vi "6220.vi"(2 "率":dbl=10.0, 3 "采样数":i32=10, 4 "timeout (s)":dbl=10.0 caption="超时(s)" format="%0.2f", 5 "error in":errorcluster caption="错误输入", 7 "stop (F)":bool caption="停止(F)", 10 "设备名":tag="PXI1Slot2") -> (14 "task out":refnum<k21> caption="任务输出", 15 "6220":cluster{"时间":timestamp, "数据":sgl[][]}, 18 "stopped":bool caption="已停止", 19 "error out":errorcluster caption="错误输出")   [LabVIEW 2014]
doc: "通过NI-DAQmx创建、编辑和运行任务。关于NI-DAQmx支持设备的完整列表，见NI-DAQ自述文件。\n\n在程序框图上放置DAQ助手Express VI，可通过DAQ助手新建任务。创建任务后，双击DAQ助手Express VI可编辑该任务。如需连续进行测量或信号生成，可将DAQ助手Express VI置于While循环内。"
uses:
  <vilib>/DAQmx/read.llb/DAQmx Read.vi
  <vilib>/DAQmx/read.llb/DAQmx Read (Analog 2D DBL NChan NSamp).vi
  <vilib>/DAQmx/miscellaneous.llb/DAQmx Fill In Error Info.vi
  <vilib>/DAQmx/configure/timing.llb/DAQmx Timing (Sample Clock).vi
  <vilib>/DAQmx/create/channels.llb/DAQmx Create Channel (AI-Voltage-Basic).vi
  <vilib>/DAQmx/create/channels.llb/DAQmx Create Channel (TEDS-AI-Voltage-Basic).vi
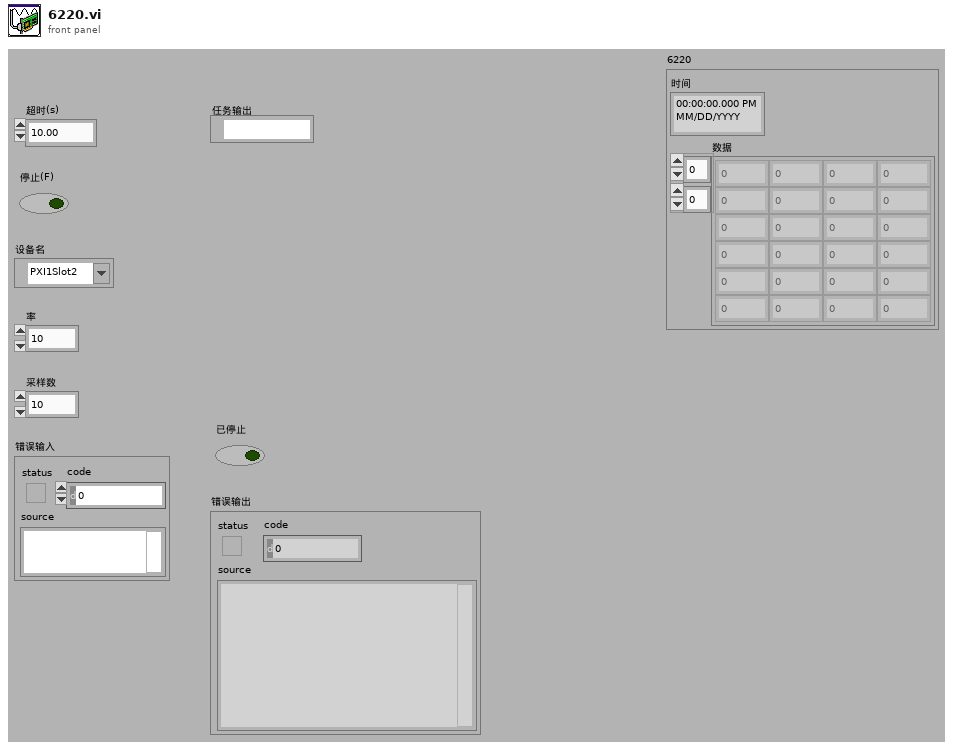
[diagram p1: front panel]
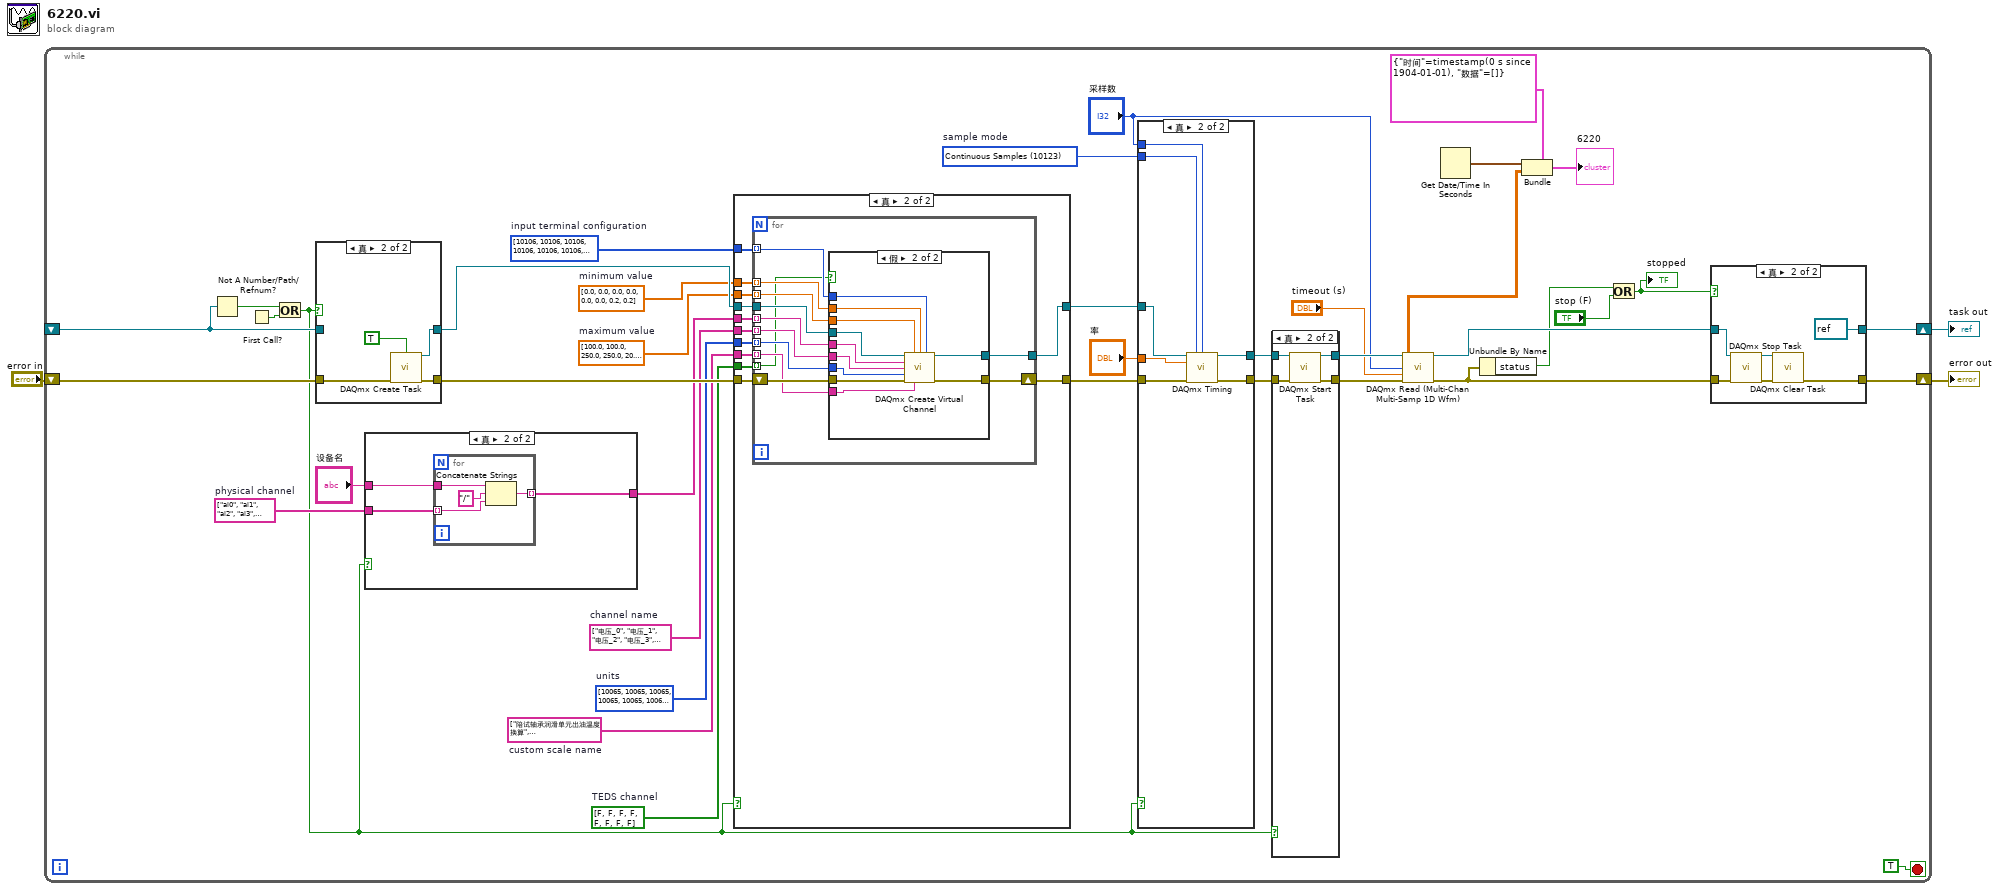
[diagram p0: block diagram]
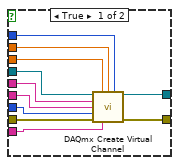
[diagram p6: hidden frame]
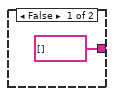
[diagram p7: hidden frame]
diagram:
  n1 = while {
    shift-right: [w14] -> w1
    shift-left: _ -> [w39]
    shift-right: [w12] -> w2
    shift-left: "error in" -> [w40]
    stop <- TRUE stop-if-true
    w22 = 10123 items=["Finite Samples"=10178, "Continuous Samples"=10123, "Hardware Timed Single Point"=12522]  # sample mode
    w26 = bool[] [FALSE, FALSE, FALSE, FALSE, FALSE, FALSE, FALSE, FALSE]  # TEDS channel
    w27 = string[] ["陪试轴承润滑单元出油温度换算", "陪试轴承润滑单元出油温度换算", "轴承外圈温度换算", "轴承外圈温度换算", "摩擦力换算", "摩擦力换算", "油缸力换算", "油缸力换算"]  # custom scale name
    w28 = i32[] [10065, 10065, 10065, 10065, 10065, 10065, 10065, 10065] items=["Volts"=10348, "From TEDS"=12516, "From Custom Scale"=10065]  # units
    w29 = string[] ["电压_0", "电压_1", "电压_2", "电压_3", "电压_4", "电压_5", "电压_6", "电压_7"]  # channel name
    w31 = dbl[] [100.0, 100.0, 250.0, 250.0, 20.0, 20.0, 7.0, 7.0]  # maximum value
    w32 = dbl[] [0.0, 0.0, 0.0, 0.0, 0.0, 0.0, 0.2, 0.2]  # minimum value
    w33 = i32[] [10106, 10106, 10106, 10106, 10106, 10106, 10106, 10106] items=["default"=-1, "RSE"=10083, "NRSE"=10078, "Differential"=10106, "Pseudodifferential"=12529]  # input terminal configuration
    w36 = string[] ["ai0", "ai1", "ai2", "ai3", "ai4", "ai5", "ai6", "ai7"]  # physical channel
    n2 = Not A Number/Path/Refnum?(number/path/refnum=w39) -> (NaN/Path/Refnum?=w38:bool)
    n3 = First Call?() -> (First Call?: T/F=w41:bool)
    n4 = Or(x=w38, y=w41) -> (x .or. y?=w21:bool)
    n5 = case "条件结构" shown="真" w21 {
      tunnel: [w123 w127] -> w35
      tunnel: w39 -> [w123 _]
      tunnel: [w122 w126] -> w34
      tunnel: w40 -> [w122 w124]
      frame False {
      }
      frame True {
        n6 = call <vilib>:"DAQmx Create Task.vi"("auto cleanup"=TRUE, "error in"=w124) -> ("task out"=w127:refnum<k21>, "error out"=w126:errorcluster)  [unwired: 12 in]
      }
    }
    n7 = case "条件结构" shown="真" w21 {
      tunnel: [string[] [] w117] -> w30
      tunnel: "设备名" -> [_ w116]
      tunnel: w36 -> [_ w115]
      frame False {
      }
      frame True {
        n8 = for "For循环" {
          tunnel: [w121] -> w117 mode=indexing
          tunnel: w116 -> [w120]
          tunnel: w115 -> [w118] mode=indexing
          n9 = Concatenate Strings(w120, "/" ("string"), w118) -> (w121:string)
        }
      }
    }
    n10 = case "条件结构" shown="真" w21 {
      tunnel: [w67 w77] -> w25
      tunnel: w35 -> [w67 w79]
      tunnel: [w66 w76] -> w24
      tunnel: w34 -> [w66 w78]
      tunnel: w33 -> [_ w75]
      tunnel: w32 -> [_ w74]
      tunnel: w31 -> [_ w73]
      tunnel: w30 -> [_ w72]
      tunnel: w29 -> [_ w71]
      tunnel: w28 -> [_ w70]
      tunnel: w27 -> [_ w69]
      tunnel: w26 -> [_ w68]
      frame False {
      }
      frame True {
        n11 = for "For循环" {
          tunnel: w79 -> [w91]
          tunnel: [w89] -> w77
          tunnel: w75 -> [w87] mode=indexing
          tunnel: w74 -> [w86] mode=indexing
          tunnel: w73 -> [w85] mode=indexing
          tunnel: w72 -> [w84] mode=indexing
          tunnel: w71 -> [w83] mode=indexing
          tunnel: w70 -> [w82] mode=indexing
          tunnel: w69 -> [w81] mode=indexing
          shift-right: [w88] -> w76
          shift-left: w78 -> [w90]
          tunnel: w68 -> [w80] mode=indexing
          n12 = case "条件结构" shown="假" w80 {
            tunnel: w91 -> [w102 w113]
            tunnel: w90 -> [w101 w112]
            tunnel: [w100 w111] -> w89
            tunnel: [w99 w110] -> w88
            tunnel: w87 -> [w98 w109]
            tunnel: w86 -> [w97 w108]
            tunnel: w85 -> [w96 w107]
            tunnel: w84 -> [w95 w106]
            tunnel: w83 -> [w94 w105]
            tunnel: w82 -> [w93 w104]
            tunnel: w81 -> [w92 w103]
            frame True {
              n13 = call-poly <vilib>:"DAQmx Create Virtual Channel.vi"("task in"=w102, "maximum value"=w96, "minimum value"=w97, "input terminal configuration"=w98, "physical channels"=w95, "name to assign"=w94, "units"=w93, "error in"=w101, "custom scale name"=w92) -> ("task out"=w100:refnum<k21>, "error out"=w99:errorcluster)  [unwired: 5 in]
            }
            frame False {
              n14 = call-poly <vilib>:"DAQmx Create Virtual Channel.vi"("task in"=w113, "maximum value"=w107, "minimum value"=w108, "input terminal configuration"=w109, "physical channels"=w106, "name to assign"=w105, "units"=w104, "error in"=w112, "custom scale name"=w103) -> ("task out"=w111:refnum<k21>, "error out"=w110:errorcluster)  [unwired: 5 in]
            }
          }
        }
      }
    }
    n15 = case "条件结构" shown="真" w21 {
      tunnel: [w58 w60] -> w20
      tunnel: w25 -> [w58 w63]
      tunnel: [w57 w59] -> w19
      tunnel: w24 -> [w57 w61]
      tunnel: "采样数" -> [_ w65]
      tunnel: w22 -> [_ w64]
      tunnel: "率" -> [_ w62]
      frame False {
      }
      frame True {
        n16 = call-poly <vilib>:"DAQmx Timing.vi"("task/channels in"=w63, "sample mode"=w64, "samples per channel"=w65, "rate"=w62, "error in"=w61) -> ("task out"=w60:refnum<k21>, "error out"=w59:errorcluster)  [unwired: 9 in]
      }
    }
    n17 = case "条件结构" shown="真" w21 {
      tunnel: [w52 w55] -> w18
      tunnel: w20 -> [w52 w56]
      tunnel: [w51 w53] -> w17
      tunnel: w19 -> [w51 w54]
      frame False {
      }
      frame True {
        n18 = call <vilib>:"DAQmx Start Task.vi"("task/channels in"=w56, "error in"=w54) -> ("task out"=w55:refnum<k21>, "error out"=w53:errorcluster)  [unwired: 12 in]
      }
    }
    n19 = call-poly "DAQmx Read (Multi-Chan Multi-Samp 1D Wfm).vi"("task/channels in"=w18, "number of samples per channel"="采样数", "timeout"="timeout (s)", "error in"=w17) -> ("task out"=w13:refnum<k21>, "data"=w6:dbl[][], "error out"=w11:errorcluster)  [unwired: 9 in]
    n20 = Get Date/Time In Seconds() -> (seconds since 1Jan1904=w7:timestamp)
    n21 = Unbundle By Name(w11) -> ("status"=w10:bool)
    n22 = Bundle(cluster=cluster{"时间":timestamp, "数据":sgl[][]} {"时间"=timestamp(0 s since 1904-01-01), "数据"=[]}, "时间"=w7, "数据"=w6) -> (→"6220":cluster{"时间":timestamp, "数据":sgl[][]})
    n23 = Or(x=w10, y="stop (F)") -> (x .or. y?=w8:bool)
    "stopped" <- w8
    n24 = case "条件结构" shown="真" w8 {
      tunnel: [w44 refnum<k21> refnum ("task in")] -> w14
      tunnel: w13 -> [w44 w50]
      tunnel: [w43 w47] -> w12
      tunnel: w11 -> [w43 w49]
      frame False {
      }
      frame True {
        n25 = call <vilib>:"DAQmx Stop Task.vi"("task/channels in"=w50, "error in"=w49) -> ("task out"=w46:refnum<k21>, "error out"=w48:errorcluster)  [unwired: 12 in]
        n26 = call <vilib>:"DAQmx Clear Task.vi"("task in"=w46, "error in"=w48) -> ("error out"=w47:errorcluster)  [unwired: 13 in]
      }
    }
  }
  "error out" <- w2
  "task out" <- w1
